vi "Read Dialog Clusters.vi"(11 "Module Cluster Refs":refnum<vi>[](array[refnum])) -> (3 "TestSequence":T1[](array[typedef]))   [LabVIEW 2017]
doc: "convert the contents of UI objects into a data structure of a seqeunce that can be executed."
uses:
  TestStep-StepType.ctl
  TestStepTypes.ctl
  RF Direction.ctl
  PolarizationSelect.ctl
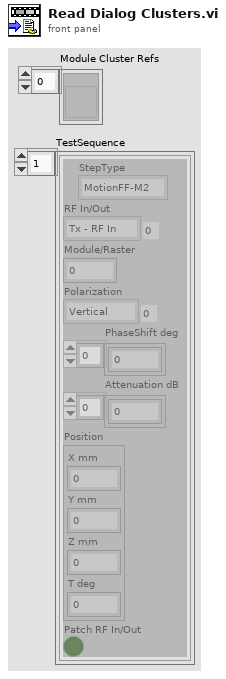
[diagram p1: front panel]
types:
  T1 = typedef "TestStep-StepType.ctl" = cluster{"StepType":T2, "RF In/Out":T3, "Module/Raster":i32, "Polarization":T4, "PhaseShift deg":dbl[], "Attenuation dB":dbl[], "Position":cluster{"X mm":dbl, "Y mm":dbl, "Z mm":dbl, "T deg":dbl}, "Patch RF In/Out":bool}
  T2 = typedef "TestStepTypes.ctl" = enum16{"MotionFF-M2", "Motion", "SweepTest", "RasterTest", "Finish", "64ModuleCfg"}
  T3 = typedef "RF Direction.ctl" = enum16{"Tx - RF In", "Rx - RF Out"}
  T4 = typedef "PolarizationSelect.ctl" = enum16{"Vertical", "Horizontal"}
  T5 = enum16{"Patch", "Motion", "SweepTest", "RasterTest", "Finish"}
  T6 = cluster{"RF In/Out":T3, "Module/Raster":i32, "Polarization":T4, "Test":T1}
  T7 = cluster{"RF In/Out":T3, "Module/Raster":i32, "Polarization":T4, "Test":T1}[]
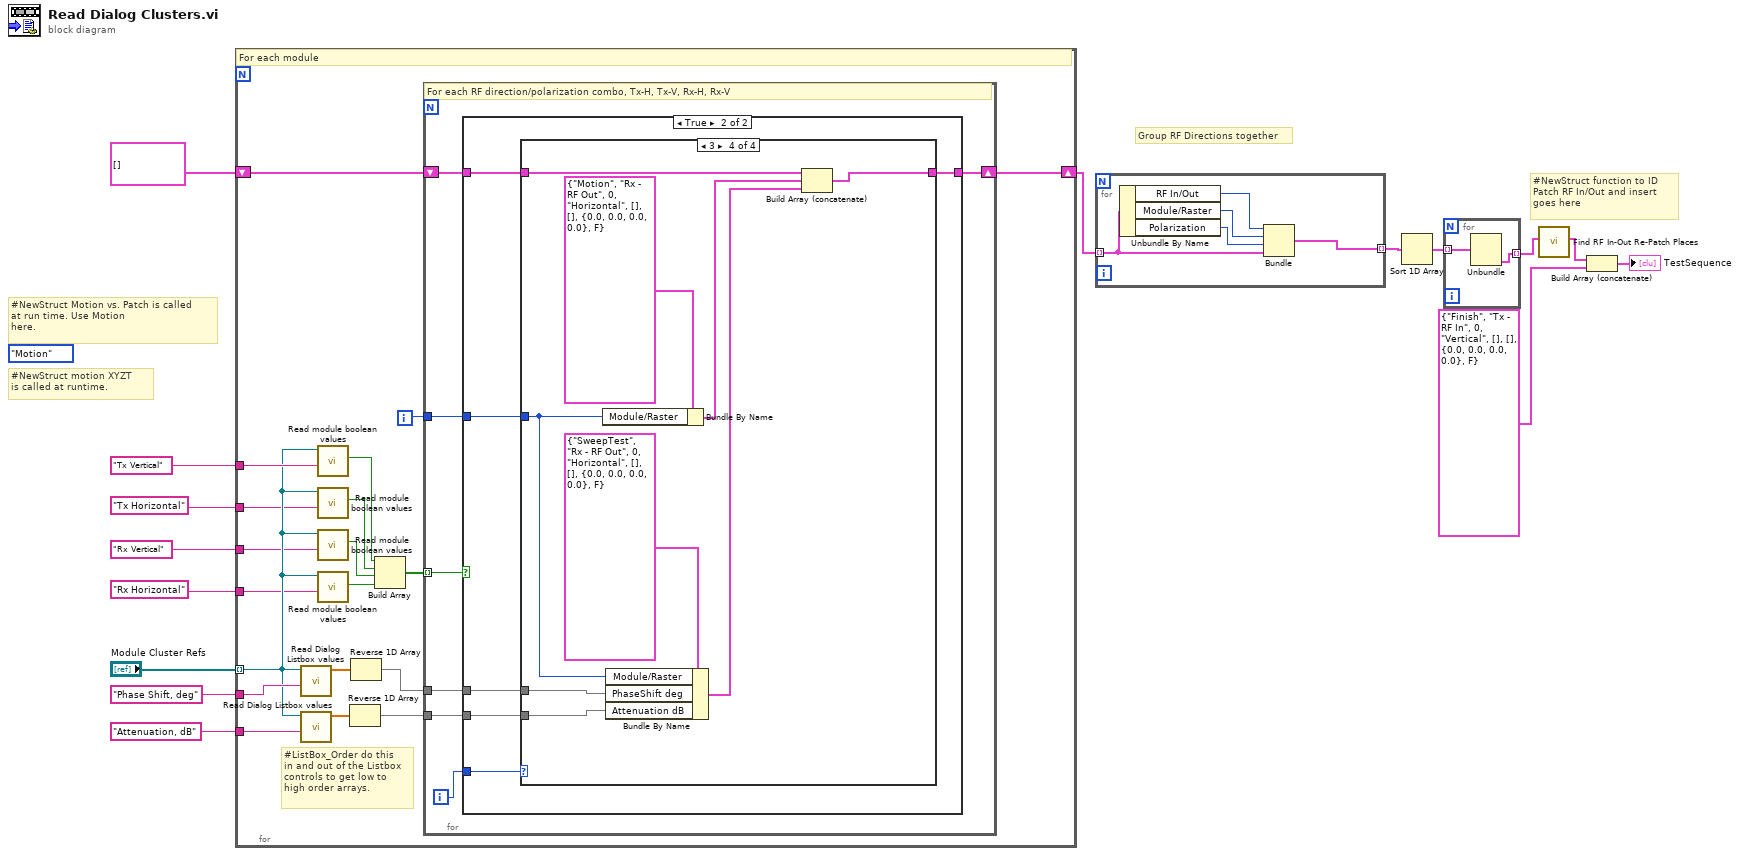
[diagram p0: block diagram]
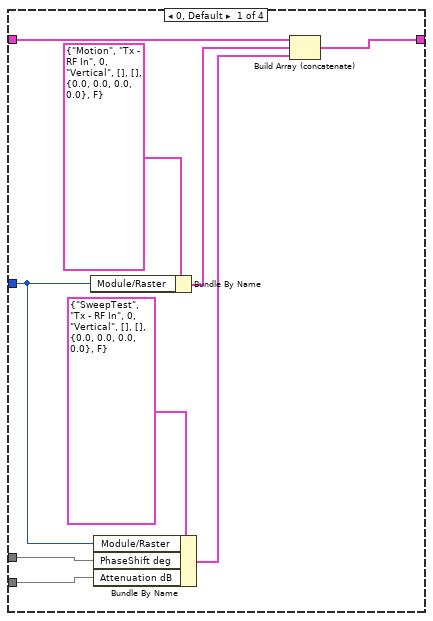
[diagram p3: hidden frame]
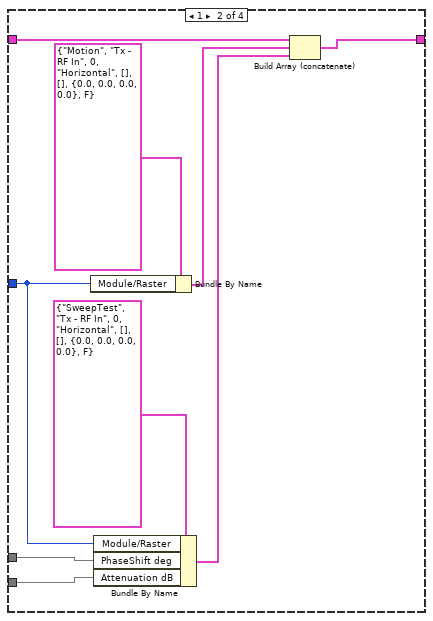
[diagram p4: hidden frame]
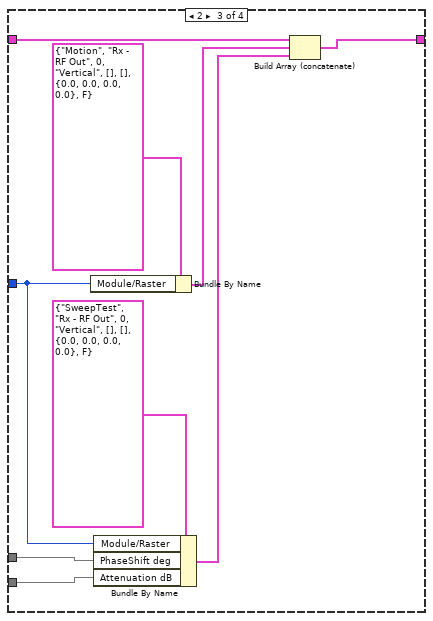
[diagram p5: hidden frame]
diagram:
  (unwired) T5."Motion" ("StepType")
  # "#NewStruct motion XYZT\nis called at runtime."
  # "#NewStruct function to ID\nPatch RF In/Out and insert\ngoes here"
  # "#NewStruct Motion vs. Patch is called\nat run time. Use Motion\nhere."
  # "Group RF Directions together"
  n1 = for {
    shift-right: [w27] -> w3
    shift-left: T1[] [] ("TestSequence") -> [w28]
    tunnel: "Module Cluster Refs" -> [w21] mode=indexing
    tunnel: "Phase Shift, deg" ("Label.Text") -> [w34]
    tunnel: "Attenuation, dB" ("Label.Text") -> [w33]
    tunnel: "Tx Vertical" ("Label.Text") -> [w25]
    tunnel: "Tx Horizontal" ("Label.Text") -> [w20]
    tunnel: "Rx Vertical" ("Label.Text") -> [w19]
    tunnel: "Rx Horizontal" ("Label.Text") -> [w18]
    i -> [w29]
    # "#ListBox_Order do this\nin and out of the Listbox\ncontrols to get low to\nhigh order arrays."
    # "For each module"
    n2 = call "Read Dialog Listbox values.vi"("Label.Text"=w34, "module ref"=w21) -> ("Values"=w31:dbl[])  [unwired: 8 in, 1 out]
    n3 = call "Read Dialog Listbox values.vi"("Label.Text"=w33, "module ref"=w21) -> ("Values"=w30:dbl[])  [unwired: 8 in, 1 out]
    n4 = call "Read module boolean values.vi"("Label.Text"=w25, "module ref"=w21) -> ("data"=w26:bool)  [unwired: 9 in]
    n5 = call "Read module boolean values.vi"("Label.Text"=w20, "module ref"=w21) -> ("data"=w23:bool)  [unwired: 9 in]
    n6 = call "Read module boolean values.vi"("Label.Text"=w19, "module ref"=w21) -> ("data"=w22:bool)  [unwired: 9 in]
    n7 = call "Read module boolean values.vi"("Label.Text"=w18, "module ref"=w21) -> ("data"=w24:bool)  [unwired: 9 in]
    n8 = Reverse 1D Array(array=w30) -> (reversed array=w16:dbl[])
    n9 = Reverse 1D Array(array=w31) -> (reversed array=w17:dbl[])
    n10 = Build Array(w26, w23, w22, w24) -> (w32:bool[])
    n11 = for {
      tunnel: w32 -> [w37] mode=indexing
      tunnel: w17 -> [w40]
      tunnel: w16 -> [w39]
      tunnel: w29 -> [w38]
      shift-right: [w35] -> w27
      shift-left: w28 -> [w36]
      i -> [w41]
      # "For each RF direction/polarization combo, Tx-H, Tx-V, Rx-H, Rx-V"
      n12 = case shown="True" w37 {
        tunnel: w41 -> [_ w48]
        tunnel: w40 -> [_ w44]
        tunnel: w39 -> [_ w43]
        tunnel: w38 -> [_ w47]
        tunnel: w36 -> [w42 w46]
        tunnel: [w42 w45] -> w35
        frame False {
          # "no test"
        }
        frame True {
          n13 = case shown="3" w48 {
            tunnel: w44 -> [w56 w65 w74 w83]
            tunnel: w43 -> [w55 w64 w73 w82]
            tunnel: w47 -> [w50 w59 w68 w77]
            tunnel: w46 -> [w53 w62 w71 w80]
            tunnel: [w49 w58 w67 w76] -> w45
            frame 0, Default {
              n14 = Bundle By Name(cluster=T1 {"StepType"=enum."Motion", "RF In/Out"=enum."Tx - RF In", "Module/Raster"=0, "Polarization"=enum."Vertical", "PhaseShift deg"=[], "Attenuation dB"=[], "Position"={"X mm"=0.0, "Y mm"=0.0, "Z mm"=0.0, "T deg"=0.0}, "Patch RF In/Out"=FALSE} ("Test"), "Module/Raster"=w50) -> (w52:T1)
              n15 = Bundle By Name(cluster=T1 {"StepType"=enum."SweepTest", "RF In/Out"=enum."Tx - RF In", "Module/Raster"=0, "Polarization"=enum."Vertical", "PhaseShift deg"=[], "Attenuation dB"=[], "Position"={"X mm"=0.0, "Y mm"=0.0, "Z mm"=0.0, "T deg"=0.0}, "Patch RF In/Out"=FALSE} ("Test"), "Module/Raster"=w50, "PhaseShift deg"=w56, "Attenuation dB"=w55) -> (w51:T1)
              n16 = Build Array (concatenate)(w53, w52, w51) -> (w49:T1[])
            }
            frame 1 {
              n17 = Bundle By Name(cluster=T1 {"StepType"=enum."Motion", "RF In/Out"=enum."Tx - RF In", "Module/Raster"=0, "Polarization"=enum."Horizontal", "PhaseShift deg"=[], "Attenuation dB"=[], "Position"={"X mm"=0.0, "Y mm"=0.0, "Z mm"=0.0, "T deg"=0.0}, "Patch RF In/Out"=FALSE} ("Test"), "Module/Raster"=w59) -> (w61:T1)
              n18 = Bundle By Name(cluster=T1 {"StepType"=enum."SweepTest", "RF In/Out"=enum."Tx - RF In", "Module/Raster"=0, "Polarization"=enum."Horizontal", "PhaseShift deg"=[], "Attenuation dB"=[], "Position"={"X mm"=0.0, "Y mm"=0.0, "Z mm"=0.0, "T deg"=0.0}, "Patch RF In/Out"=FALSE} ("Test"), "Module/Raster"=w59, "PhaseShift deg"=w65, "Attenuation dB"=w64) -> (w60:T1)
              n19 = Build Array (concatenate)(w62, w61, w60) -> (w58:T1[])
            }
            frame 2 {
              n20 = Bundle By Name(cluster=T1 {"StepType"=enum."Motion", "RF In/Out"=enum."Rx - RF Out", "Module/Raster"=0, "Polarization"=enum."Vertical", "PhaseShift deg"=[], "Attenuation dB"=[], "Position"={"X mm"=0.0, "Y mm"=0.0, "Z mm"=0.0, "T deg"=0.0}, "Patch RF In/Out"=FALSE} ("Test"), "Module/Raster"=w68) -> (w70:T1)
              n21 = Bundle By Name(cluster=T1 {"StepType"=enum."SweepTest", "RF In/Out"=enum."Rx - RF Out", "Module/Raster"=0, "Polarization"=enum."Vertical", "PhaseShift deg"=[], "Attenuation dB"=[], "Position"={"X mm"=0.0, "Y mm"=0.0, "Z mm"=0.0, "T deg"=0.0}, "Patch RF In/Out"=FALSE} ("Test"), "Module/Raster"=w68, "PhaseShift deg"=w74, "Attenuation dB"=w73) -> (w69:T1)
              n22 = Build Array (concatenate)(w71, w70, w69) -> (w67:T1[])
            }
            frame 3 {
              n23 = Bundle By Name(cluster=T1 {"StepType"=enum."Motion", "RF In/Out"=enum."Rx - RF Out", "Module/Raster"=0, "Polarization"=enum."Horizontal", "PhaseShift deg"=[], "Attenuation dB"=[], "Position"={"X mm"=0.0, "Y mm"=0.0, "Z mm"=0.0, "T deg"=0.0}, "Patch RF In/Out"=FALSE} ("Test"), "Module/Raster"=w77) -> (w79:T1)
              n24 = Bundle By Name(cluster=T1 {"StepType"=enum."SweepTest", "RF In/Out"=enum."Rx - RF Out", "Module/Raster"=0, "Polarization"=enum."Horizontal", "PhaseShift deg"=[], "Attenuation dB"=[], "Position"={"X mm"=0.0, "Y mm"=0.0, "Z mm"=0.0, "T deg"=0.0}, "Patch RF In/Out"=FALSE} ("Test"), "Module/Raster"=w77, "PhaseShift deg"=w83, "Attenuation dB"=w82) -> (w78:T1)
              n25 = Build Array (concatenate)(w80, w79, w78) -> (w76:T1[])
            }
          }
        }
      }
    }
  }
  n26 = for {
    tunnel: w3 -> [w89] mode=indexing
    tunnel: [w88] -> w4 mode=indexing
    n27 = Unbundle By Name(w89) -> ("RF In/Out"=w87:T3, "Module/Raster"=w86:i32, "Polarization"=w85:T4)
    n28 = Bundle("RF In/Out"=w87, "Module/Raster"=w86, "Polarization"=w85, "Test"=w89) -> (w88:T6)  [unwired: 1 in]
  }
  n29 = Sort 1D Array(array=w4) -> (sorted array=w12:T7)
  n30 = for {
    tunnel: w12 -> [w91] mode=indexing
    tunnel: [w90] -> w2 mode=indexing
    n31 = Unbundle(w91) -> ("Test"=w90:T1)  [unwired: 3 out]
  }
  n32 = call "Find RF In-Out Re-Patch Places.vi"("TestSequence"=w2) -> ("TestSequence out"=w1:T1[])  [unwired: 10 in]
  n33 = Build Array (concatenate)(w1, T1 {"StepType"=enum."Finish", "RF In/Out"=enum."Tx - RF In", "Module/Raster"=0, "Polarization"=enum."Vertical", "PhaseShift deg"=[], "Attenuation dB"=[], "Position"={"X mm"=0.0, "Y mm"=0.0, "Z mm"=0.0, "T deg"=0.0}, "Patch RF In/Out"=FALSE} ("Test")) -> (→"TestSequence":T1[])
